vi "Color Changing FS.vi"(0 "Feature In":string="FeatureScript 1247;\nimport(path : \"onshape/std/geometry.fs\", version : \"1247.0\");\n\nannotation { \"Feature Type Name\" : \"LabVIEW Feature\" }\nexport const myFeature = defineFeature(function(context is Context, id is Id, definition is map)\n    precondition\n    {\n        // Define the parameters of the feature type\n    }\n    {\n        // Define the function's action\n\nvar sketch1 = newSketch(context, id + \"sketch1\", {\n                \"sketchPlane\" : qCreatedBy(makeId(\"Top\"), EntityType.FACE)\n        });\n        // Create sketch entities here\n        skRectangle(sketch1, \"rectangle1\", {\n                \"firstCorner\" : vector(0, 0) * inch,\n                \"secondCorner\" : vector(3, 4) * inch\n        });\n        \n        skSolve(sketch1);\n    });", 4 "Cuboid":T1={"Point 1"={"x"=0.0, "y"=0.0, "z"=0.0}, "Point 2"={"x"=1.0, "y"=1.0, "z"=1.0}, "Point 3"={"x"=1.0, "y"=1.0, "z"=1.0}}, 5 "Body #":i32=1) -> (14 "Feature Out":string="FeatureScript 1247;\nimport(path : \"onshape/std/geometry.fs\", version : \"1247.0\");\n\nannotation { \"Feature Type Name\" : \"LVFeat1\" }\nexport const myFeature = defineFeature(function(context is Context, id is Id, definition is map)\n    precondition\n    {\n        // Define the parameters of the feature type\n    }\n    {\n        // Define the function's action\n       fEllipsoid(context, id + \"ellipsoid1\", {\n                \"center\" : vector(5, 0, 0) * inch,\n                \"radius\" : vector(3, 3, 3) * inch,\n        });\n\nvar sketch1 = newSketch(context, id + \"sketch1\", {\n                \"sketchPlane\" : qCreatedBy(makeId(\"Top\"), EntityType.FACE)\n        });\n        // Create sketch entities here\n        skRectangle(sketch1, \"rectangle1\", {\n                \"firstCorner\" : vector(0, 0) * inch,\n                \"secondCorner\" : vector(3, 4) * inch\n        });\n        \n        skSolve(sketch1);\n    });")   [LabVIEW 2020]
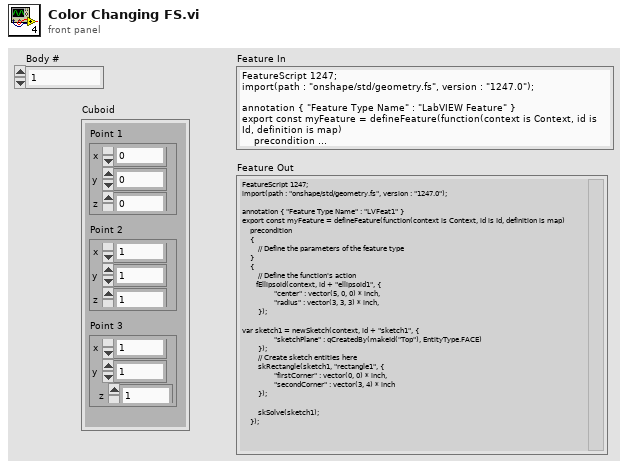
[diagram p1: front panel]
types:
  T1 = cluster{"Point 1":cluster{"x":dbl, "y":dbl, "z":dbl}, "Point 2":cluster{"x":dbl, "y":dbl, "z":dbl}, "Point 3":cluster{"x":dbl, "y":dbl, "z":dbl}}
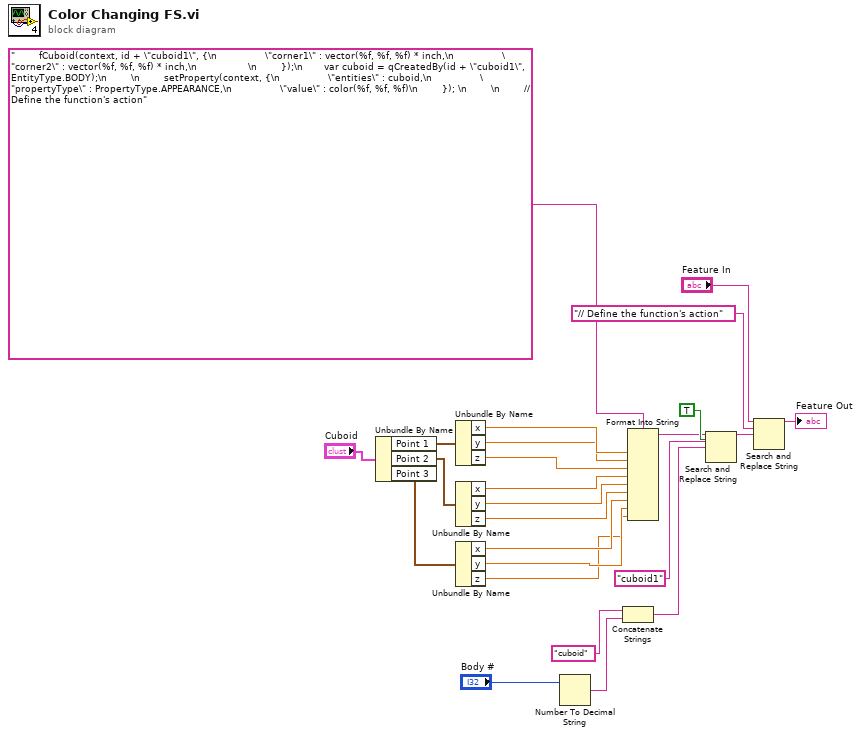
[diagram p0: block diagram]
diagram:
  n1 = Unbundle By Name("Cuboid") -> ("Point 1"=w20:cluster{"x":dbl, "y":dbl, "z":dbl}, "Point 2"=w19:cluster{"x":dbl, "y":dbl, "z":dbl}, "Point 3"=w1:cluster{"x":dbl, "y":dbl, "z":dbl})
  n2 = Unbundle By Name(w20) -> ("x"=w12:dbl, "y"=w11:dbl, "z"=w10:dbl)
  n3 = Unbundle By Name(w19) -> ("x"=w9:dbl, "y"=w8:dbl, "z"=w7:dbl)
  n4 = Unbundle By Name(w1) -> ("x"=w4:dbl, "y"=w3:dbl, "z"=w2:dbl)
  n5 = Number To Decimal String(number="Body #") -> (decimal integer string=w14:string)  [unwired: 1 in]
  n6 = Concatenate Strings("cuboid" ("regular expression"), w14) -> (w15:string)
  n7 = Format Into String(format string="        fCuboid(context, id + \"cuboid1\", {\n                \"corner1\" : vector(%f, %f, %f) * inch,\n                \"corner2\" : vector(%f, %f, %f) * inch,\n                 \n        });\n       var cuboid = qCreatedBy(id + \"cuboid1\", EntityType.BODY);\n        \n        setProperty(context, {\n                \"entities\" : cuboid,\n                \"propertyType\" : PropertyType.APPEARANCE,\n                \"value\" : color(%f, %f, %f)\n        }); \n        \n        // Define the function's action" ("search string"), w12, w11, w10, w9, w8, w7, w4, w3, w2) -> (resulting string=w6:string)  [unwired: 2 in, 1 out]
  n8 = Search and Replace String(replace all?=TRUE ("replace all? (F)"), input string=w6, search string="cuboid1" ("regular expression"), replace string=w15) -> (result string=w13:string)  [unwired: 4 in, 3 out]
  n9 = Search and Replace String(input string="Feature In", search string="// Define the function's action", replace string=w13) -> (result string=→"Feature Out":string)  [unwired: 5 in, 3 out]
